vi "TestCOMMultiFuncall.vi"() -> ()   [LabVIEW 2012]
panel:
  out "cuberoot":dbl
  out "squareroot":dbl
  out "cube":dbl
  out "square":dbl
  in  "cbrtinput":dbl
  in  "sqrtinput":dbl
  in  "cbinput":dbl
  in  "sqinput":dbl
  in  "myunitedcom.IRoot":refnum<k7>
  in  "myunitedcom.IPower":refnum<k7>
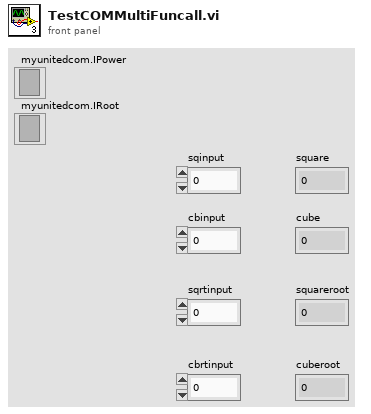
[diagram p1: front panel]
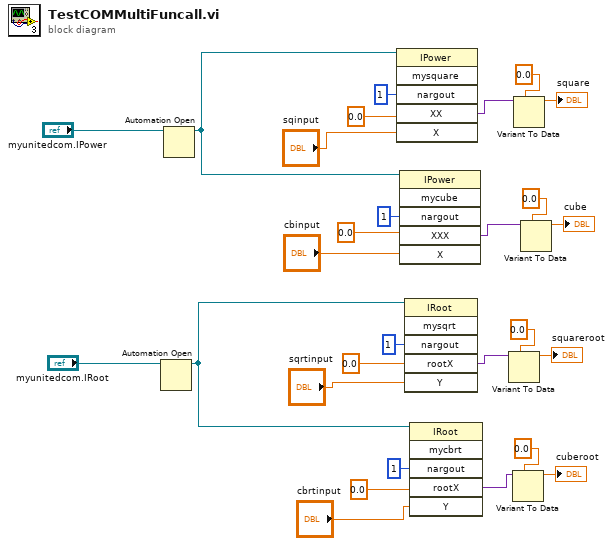
[diagram p0: block diagram]
diagram:
  n1 = Automation Open(Automation Refnum="myunitedcom.IRoot") -> (Automation Refnum=w25:refnum<k7>)  [unwired: 3 in, 1 out]
  n2 = Automation Open(Automation Refnum="myunitedcom.IPower") -> (Automation Refnum=w26:refnum<k7>)  [unwired: 3 in, 1 out]
  n3 = invoke class="IPower" method="mysquare"(reference=w26, "nargout"=1, "XX"=0.0, "X"="sqinput") -> ("XX"=w4:variant)  [unwired: 2 in, 5 out]
  n4 = invoke class="IPower" method="mycube"(reference=w26, "nargout"=1, "XXX"=0.0, "X"="cbinput") -> ("XXX"=w3:variant)  [unwired: 2 in, 5 out]
  n5 = invoke class="IRoot" method="mysqrt"(reference=w25, "nargout"=1, "rootX"=0.0, "Y"="sqrtinput") -> ("rootX"=w2:variant)  [unwired: 2 in, 5 out]
  n6 = invoke class="IRoot" method="mycbrt"(reference=w25, "nargout"=1, "rootX"=0.0, "Y"="cbrtinput") -> ("rootX"=w1:variant)  [unwired: 2 in, 5 out]
  n7 = Variant To Data(type=0.0, Variant=w2) -> (data=→"squareroot":dbl)  [unwired: 1 in, 1 out]
  n8 = Variant To Data(type=0.0, Variant=w1) -> (data=→"cuberoot":dbl)  [unwired: 1 in, 1 out]
  n9 = Variant To Data(type=0.0, Variant=w4) -> (data=→"square":dbl)  [unwired: 1 in, 1 out]
  n10 = Variant To Data(type=0.0, Variant=w3) -> (data=→"cube":dbl)  [unwired: 1 in, 1 out]
